vi "ProcessBotMove.vi"(7 "BotData":T2, 8 "error in (no error)":errorcluster, 9 "Timeout (ms)":i32=1000, 10 "GameState":T3, 11 "Bot in":T5) -> (0 "error out":errorcluster, 1 "TimedOut?":bool, 2 "NewPlayerPosition":T4, 3 "Bot out":T5, 5 "Move":T1)   [LabVIEW 2015, in "TronVIEWGameUtilities.lvlib"]
uses:
  TronVIEWGameUtilities.lvlib
  TronVIEWBotAPI/BotVIRefnum.ctl
  TronviewGame/Board/Position.ctl
  TronVIEWBotAPI/GameState.ctl
  TronVIEWBotAPI/BotData.ctl
  TronVIEWBotAPI/MovementDirection.ctl
  TronviewGame/Board/Board.lvclass
  TronVIEWBotAPI/TronVIEWBotAPI.lvlib
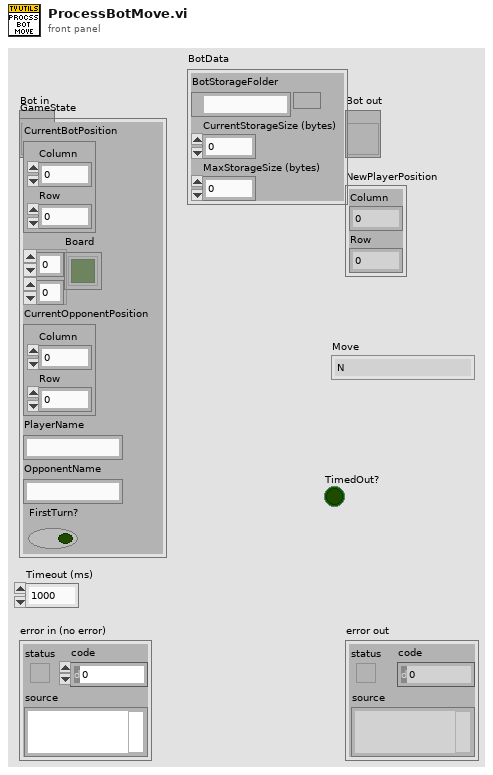
[diagram p1: front panel]
types:
  T1 = typedef "TronVIEWBotAPI.lvlib/MovementDirection.ctl" = enum16{"N", "S", "W", "E"}
  T2 = typedef "TronVIEWBotAPI.lvlib/BotData.ctl" = cluster{"BotStorageFolder":path, "CurrentStorageSize (bytes)":i64, "MaxStorageSize (bytes)":i64}
  T3 = typedef "TronVIEWBotAPI.lvlib/GameState.ctl" = cluster{"CurrentBotPosition":T4, "Board":bool[][], "CurrentOpponentPosition":T4, "PlayerName":string, "OpponentName":string, "FirstTurn?":bool}
  T4 = typedef "TronviewGame.lvlib/Board.lvclass/Position.ctl" = cluster{"Column":i32, "Row":i32}
  T5 = typedef "TronVIEWBotAPI.lvlib/BotVIRefnum.ctl" = refnum<vi>
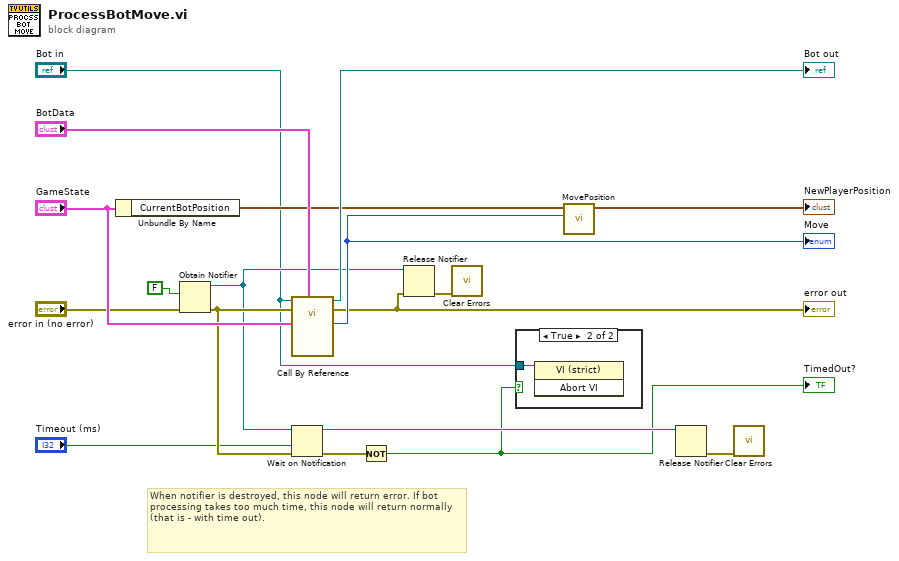
[diagram p0: block diagram]
diagram:
  # "When notifier is destroyed, this node will return error. If bot processing takes too much time, this node will return normally (that is - with time out)."
  n1 = Unbundle By Name("GameState") -> ("CurrentBotPosition"=w16:T4)
  n2 = Obtain Notifier(notification data type=FALSE, error in (no error)="error in (no error)") -> (notifier out=w10:refnum<notifier>, error out=w11:errorcluster)  [unwired: 2 in, 1 out]
  n3 = call-by-ref "?"(reference="Bot in", error in=w11, "BotData"="BotData", "GameState"="GameState") -> (reference out=→"Bot out":T5, error out=w2:errorcluster, "Move"=w15:T1)  [unwired: 8 in, 1 out]
  "error out" <- w2
  "Move" <- w15
  n4 = Wait on Notification(notifier=w10, timeout in ms (-1)="Timeout (ms)", error in (no error)=w11) -> (notifier out=w8:refnum<notifier>, error out=w5:errorcluster)  [unwired: 1 in, 2 out]
  n5 = Not(x=w5) -> (.not. x?=w4:bool)
  "TimedOut?" <- w4
  n6 = Release Notifier(notifier=w10, error in (no error)=w2) -> (error out=w1:errorcluster)  [unwired: 1 in, 2 out]
  n7 = call <vilib>:"Clear Errors.vi"("error in (no error)"=w1) -> ()  [unwired: 5 in, 2 out]
  n8 = case shown="True" w4 {
    tunnel: "Bot in" -> [_ w19]
    frame False {
    }
    frame True {
      n9 = invoke class="VI (strict)" method="Abort VI"(reference=w19) -> ()  [unwired: 2 in, 3 out]
    }
  }
  n10 = call "MovePosition.vi"("Direction"=w15, "PlayerPosition"=w16) -> ("NewPlayerPosition"=→"NewPlayerPosition":T4)  [unwired: 9 in]
  n11 = Release Notifier(notifier=w8) -> (error out=w7:errorcluster)  [unwired: 2 in, 2 out]
  n12 = call <vilib>:"Clear Errors.vi"("error in (no error)"=w7) -> ()  [unwired: 5 in, 2 out]
